vi "Transceiver Transmit.vi"(8 "error in (no error)":errorcluster, 10 "Transfer Group in":refnum<class "Transfer Group.lvclass">, 11 "Transceiver Thread in":refnum<class "Plugin Thread.lvclass">) -> (0 "error out":errorcluster, 2 "Transfer Group out":refnum<class "Transfer Group.lvclass">, 3 "Transceiver Thread out":refnum<class "Plugin Thread.lvclass">)   [LabVIEW 2017, in "DSF Core.lvlib" / "Plugin Thread.lvclass"]
uses:
  Thread/Plugin/Plugin Thread.lvclass
  Transfer Group/Transfer Group.lvclass
  Thread/Plugin/Plugin Thread.lvclass/Plugin Thread.ctl
  Transceiver.lvclass
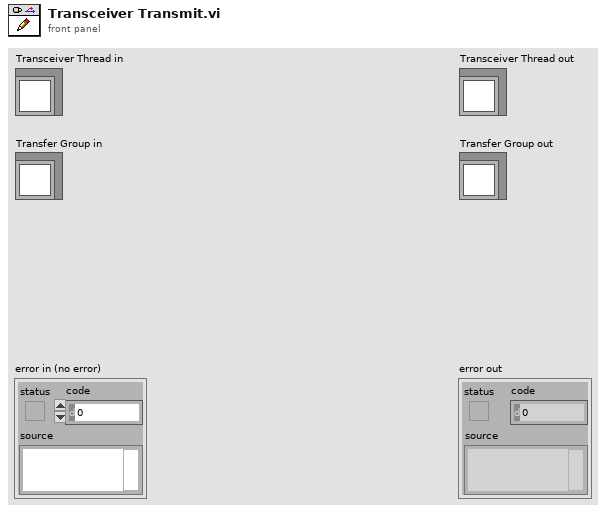
[diagram p1: front panel]
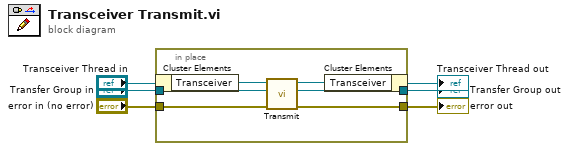
[diagram p0: block diagram]
diagram:
  n1 = in-place {
    in-place-border: "error in (no error)" -> [w12]
    in-place-border: "Transfer Group in" -> [w11]
    in-place-border: [w10] -> w3
    in-place-border: [w9] -> w2
    n2 = in-place-cluster #1("Transceiver Thread in") -> ("Transceiver"=w8:refnum<class "Transceiver.lvclass">)
    n3 = call-dynamic "Transmit.vi"("error in (no error)"=w12, "Transfer Group in"=w11, "Transceiver in"=w8) -> ("error out"=w10:errorcluster, "Transfer Group out"=w9:refnum<class "Transfer Group.lvclass">, "Transceiver out"=w7:refnum<class "Transceiver.lvclass">)  [unwired: 6 in]
    n4 = in-place-cluster #1("Transceiver"=w7) -> (→"Transceiver Thread out":refnum<class "Plugin Thread.lvclass">)
  }
  "error out" <- w3
  "Transfer Group out" <- w2
